vi "Check Broken VIs.vi"() -> ()   [LabVIEW 2020, in "PicoG-App.lvlib" / "picoG.lvclass"]
uses:
  picoG.lvclass
panel:
  out "Array 2":string[](array[string])
  out "Array":string[](array[string])
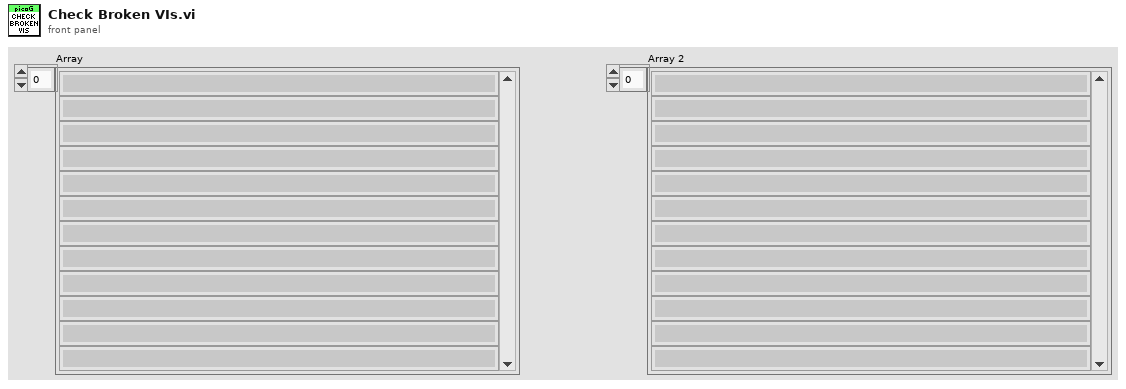
[diagram p1: front panel]
types:
  T1 = enum32{"Bad", "Idle", "Run top level", "Running"}
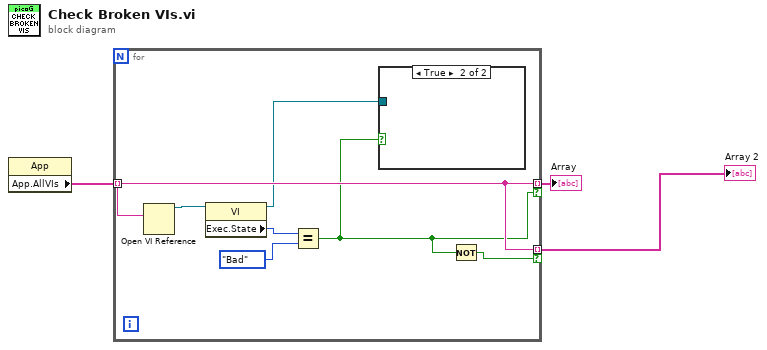
[diagram p0: block diagram]
diagram:
  n1 = property class="App"() -> ("App.AllVIs"=w3:string[])  [unwired: 2 in, 2 out]
  n2 = for {
    tunnel: w3 -> [w7] mode=indexing
    tunnel: [w7] -> w2 mode=indexing if=w4
    tunnel: [w7] -> w1 mode=indexing if=w6
    n3 = Open VI Reference(vi path=w7) -> (vi reference=w10:refnum<vi>)  [unwired: 5 in, 1 out]
    n4 = property class="VI"(reference=w10) -> (reference out=w5:refnum<vi>, "Exec.State"=w9:T1)  [unwired: 1 in, 1 out]
    n5 = Equal?(x=w9, y=T1."Bad" ("Execution:State")) -> (x = y?=w4:bool)
    n6 = case shown="True" w4 {
      tunnel: w5 -> [_ _]
      frame False {
      }
      frame True {
      }
    }
    n7 = Not(x=w4) -> (.not. x?=w6:bool)
  }
  "Array" <- w2
  "Array 2" <- w1
